vi "SetAutoShutter.vi"(8 "error in (no error)":errorcluster, 9 "Value":bool, 10 "Label":string, 11 "DemoLasers in":refnum<class "DemoLasers.lvclass">) -> (0 "error out":errorcluster, 3 "DemoLasers out":refnum<class "DemoLasers.lvclass">)   [LabVIEW 2020, in "DemoLasers.lvlib" / "DemoLasers.lvclass"]
uses:
  DemoLasers.lvclass
  Hardware Abstraction Layer/Component/Laser/Laser/Laser.lvclass
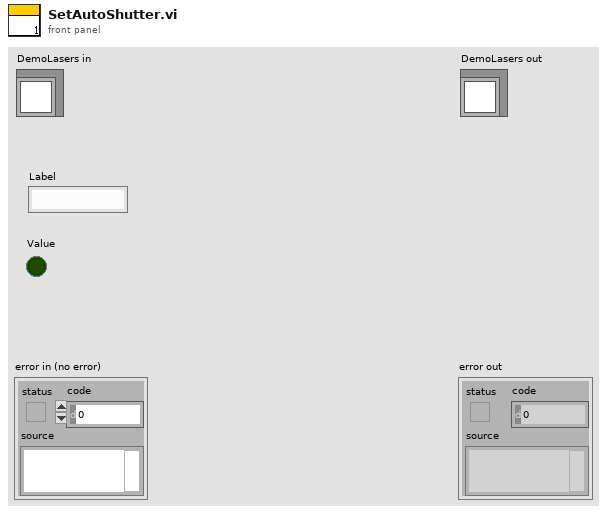
[diagram p1: front panel]
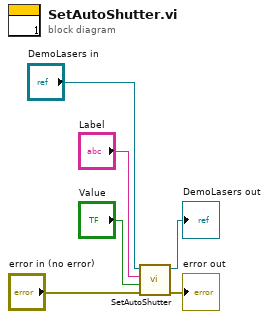
[diagram p0: block diagram]
diagram:
  n1 = call-parent "SetAutoShutter.vi"("error in (no error)"="error in (no error)", "Value"="Value", "Label"="Label", "Laser in"="DemoLasers in") -> ("error out"=→"error out":errorcluster, "Laser out"=→"DemoLasers out":refnum<class "DemoLasers.lvclass">)  [unwired: 6 in]
